vi "Write Tim Obs.vi"(8 "error in (no error)":errorcluster, 10 "Tim Obs":refnum<class "Tim File Observer.lvclass">, 11 "tCRD in":refnum<class "tCRD.lvclass">) -> (0 "error out":errorcluster, 3 "tCRD out":refnum<class "tCRD.lvclass">)   [LabVIEW 2015, in "tCRD.lvclass"]
uses:
  tCRD.lvclass
  File Observer/Tim File Observer.lvclass
  tCRD.lvclass/tCRD.ctl
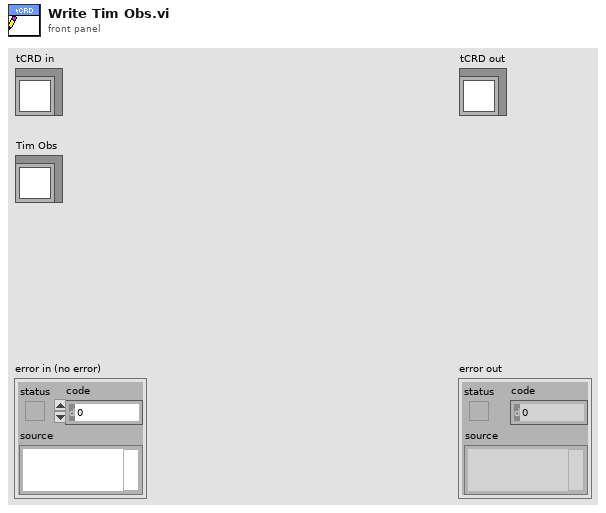
[diagram p1: front panel]
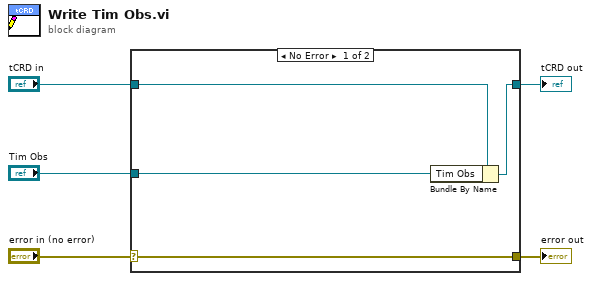
[diagram p0: block diagram]
diagram:
  n1 = case shown="No Error" "error in (no error)" {
    selector: "error in (no error)" -> [w9 w10]
    tunnel: [w9 w10] -> w4
    tunnel: [w7 w11] -> w2
    tunnel: "tCRD in" -> [w8 w11]
    tunnel: "Tim Obs" -> [w6 _]
    frame No Error {
      n2 = Bundle By Name(cluster=w8, "Tim Obs"=w6) -> (w7:refnum<class "tCRD.lvclass">)
    }
    frame Error {
    }
  }
  "error out" <- w4
  "tCRD out" <- w2
